vi "LabVIEW Coordinates to Picture Coordinates.vi"(8 "에러 입력":errorcluster, 10 "컨트롤 참조":refnum<vi>, 11 "LabVIEW 좌표계":cluster{"Horizontal":i32, "Vertical":i32}) -> (0 "에러 출력":errorcluster, 3 "그림 컨트롤 좌표계":cluster{"Horizontal":i32, "Vertical":i32})   [LabVIEW 2018]
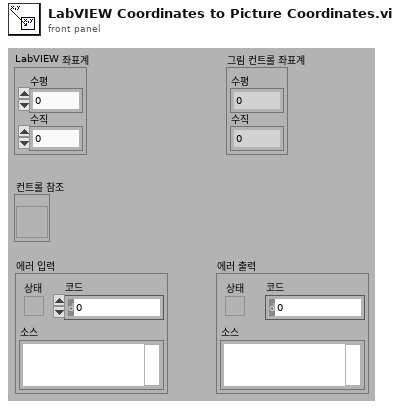
[diagram p1: front panel]
types:
  T1 = typedef "LVBoundsTypeDef.ctl" = cluster{"Width":u32, "Height":u32}
  T2 = typedef "LVPositionTypeDef.ctl" = cluster{"Left":i32, "Top":i32}
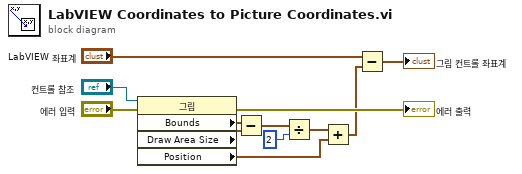
[diagram p0: block diagram]
diagram:
  n1 = property class="그림"(reference="컨트롤 참조", error in="에러 입력") -> (error out=→"에러 출력":errorcluster, "Bounds"=w3:T1, "Draw Area Size"=w4:T1, "Position"=w8:T2)  [unwired: 1 out]
  n2 = Subtract(x=w3, y=w4) -> (x-y=w6:T1)
  n3 = Divide(x=w6, y=2) -> (x/y=w7:cluster{"Width":dbl, "Height":dbl})
  n4 = Add(x=w7, y=w8) -> (x+y=w10:cluster{dbl, dbl})
  n5 = Subtract(x="LabVIEW 좌표계", y=w10) -> (x-y=→"그림 컨트롤 좌표계":cluster{dbl, dbl})
